vi "DI_parametry z kontrolki.vi"(8 "error in (no error)":errorcluster, 11 "Kanały cyfrowe in":T1) -> (0 "error out":errorcluster, 1 "Opisy out":string[](array[string]), 2 "Aktywne out":bool[](array[boolean]), 3 "Mnożniki out":dbl[](array[numeric]))   [LabVIEW 2014]
doc: "Wyodrębnia aktywne kanały cyfrowe\ni ich mnożniki"
uses:
  Kontrolki/GUI/DI_aktywacja.ctl
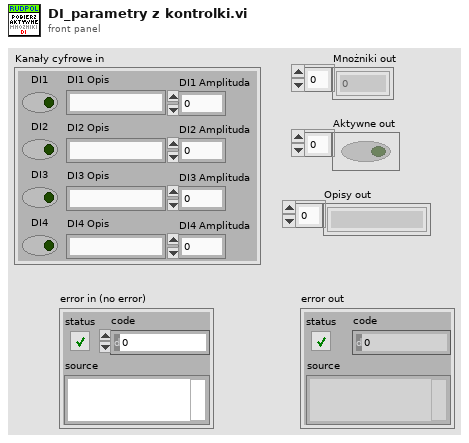
[diagram p1: front panel]
types:
  T1 = typedef "DI_aktywacja.ctl" = cluster{"DI1":bool, "DI2":bool, "DI3":bool, "DI4":bool, "DI1 Opis":string, "DI2 Opis":string, "DI3 Opis":string, "DI4 Opis":string, "DI1 Amplituda":dbl, "DI2 Amplituda":dbl, "DI3 Amplituda":dbl, "DI4 Amplituda":dbl}
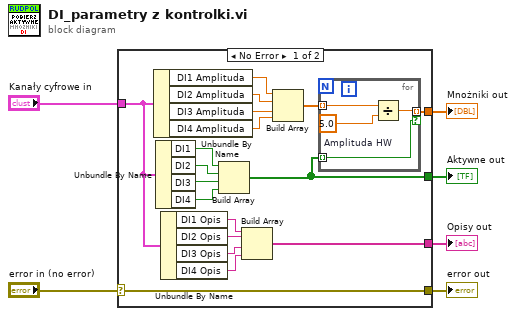
[diagram p0: block diagram]
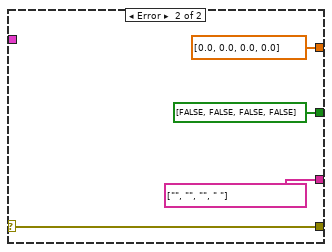
[diagram p2: hidden frame]
diagram:
  n1 = case shown="No Error" "error in (no error)" {
    selector: "error in (no error)" -> [w13 w32]
    tunnel: "Kanały cyfrowe in" -> [w8 _]
    tunnel: [w24 dbl[] [0.0, 0.0, 0.0, 0.0]] -> w5
    tunnel: [w23 bool[] [FALSE, FALSE, FALSE, FALSE]] -> w4
    tunnel: [w13 w32] -> w2
    tunnel: [w7 string[] ["", "", "", " "]] -> w1
    frame No Error {
      n2 = Unbundle By Name(w8) -> ("DI1 Amplituda"=w18:dbl, "DI2 Amplituda"=w19:dbl, "DI3 Amplituda"=w20:dbl, "DI4 Amplituda"=w21:dbl)
      n3 = Unbundle By Name(w8) -> ("DI1"=w14:bool, "DI2"=w15:bool, "DI3"=w16:bool, "DI4"=w17:bool)
      n4 = Unbundle By Name(w8) -> ("DI1 Opis"=w9:string, "DI2 Opis"=w10:string, "DI3 Opis"=w11:string, "DI4 Opis"=w12:string)
      n5 = Build Array(w14, w15, w16, w17) -> (w23:bool[])
      n6 = Build Array(w9, w10, w11, w12) -> (w7:string[])
      n7 = Build Array(w18, w19, w20, w21) -> (w22:dbl[])
      n8 = for {
        tunnel: w22 -> [w28] mode=indexing
        tunnel: w23 -> [w26] mode=indexing
        tunnel: [w27] -> w24 mode=indexing if=w26
        w25 = 5.0  # Amplituda HW
        n9 = Divide(x=w28, y=w25) -> (x/y=w27:dbl)
      }
    }
    frame Error {
    }
  }
  "Mnożniki out" <- w5
  "Aktywne out" <- w4
  "error out" <- w2
  "Opisy out" <- w1
